vi "niLvFpga_AcknowledgeIrq_USB-7846R.vi"(0 "session in":u32, 5 "IRQ Numbers":i32[](array[numeric]), 11 "error in":errorcluster) -> (4 "session out":u32, 15 "error out":errorcluster)   [LabVIEW 2020]
uses:
  <vilib>/rvi/interface/common/niFpgaWaitOnOcc.vi
  NiFpgaLv.dll
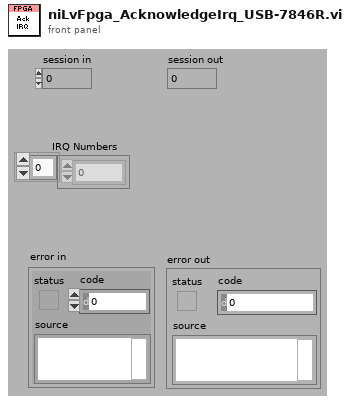
[diagram p1: front panel]
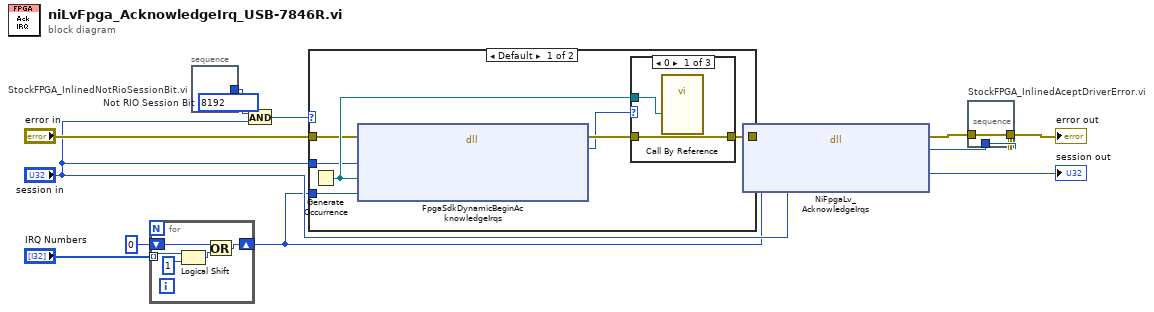
[diagram p0: block diagram]
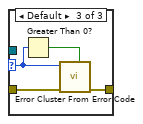
[diagram p4: hidden frame]
diagram:
  n1 = for {
    tunnel: "IRQ Numbers" -> [w16] mode=indexing
    shift-right: [w13] -> w1
    shift-left: u32 0 -> [w15]
    n2 = Logical Shift(y=w16, x=u32 1) -> (x << y=w14:u32)
    n3 = Or(x=w15, y=w14) -> (x .or. y?=w13:u32)
  }
  n4 = stacked-sequence "StockFPGA_InlinedNotRioSessionBit.vi" {
    tunnel: [w18] -> w6
    frame #0 {
      w18 = u32 8192  # Not RIO Session Bit
    }
  }
  n5 = And(x=w6, y="session in") -> (x .and. y?=w5:u32)
  n6 = case shown="Default" w5 {
    tunnel: "error in" -> [w22 w33]
    tunnel: [w21 w33] -> w3
    tunnel: "session in" -> [w20 _]
    tunnel: w1 -> [w19 _]
    frame Default {
      n7 = Generate Occurrence() -> (w25:refnum<k4>)
      n8 = dll-call lib="LabVIEW" fn="FpgaSdkDynamicBeginAcknowledgeIrqs" label="BeginAcknowledgeIrqs"(error in=w22, "session"=w20, "occurrence"=w25, "irqMask"=w19) -> (error out=w24:errorcluster, "status"=w23:i32)  [unwired: 5 in, 1 out]
      n9 = case shown="0" w23 {
        selector: w23 -> [_ _ w29]
        tunnel: [w27 w28 w31] -> w21
        tunnel: w24 -> [w27 w28 w32]
        tunnel: w25 -> [w26 _ _]
        frame 0 {
          n10 = call-by-ref "?"("occurrence"=w26) -> ()  [unwired: 16 in, 3 out]
        }
        frame -61167 {
          # "emulation case intentionally ignoring error"
        }
        frame Default {
          n11 = Greater Than 0?(x=w29) -> (x > 0?=w30:bool)
          n12 = call <vilib>:"Error Cluster From Error Code.vi"("is warning? (False)"=w30, "error in (no error)"=w32, "error code (0)"=w29) -> ("error out"=w31:errorcluster)  [unwired: 6 in]
        }
      }
    }
    frame 0 {
    }
  }
  n13 = dll-call lib="NiFpgaLv.*" fn="NiFpgaLv_AcknowledgeIrqs" label="niLvFpgaAcknowledgeIRQ"(error in=w3, "sessionID"="session in", "irqNumberMask"=w1) -> (error out=w11:errorcluster, "status"=w10:i32, "sessionID"=→"session out":u32)  [unwired: 3 in, 1 out]
  n14 = stacked-sequence "StockFPGA_InlinedAceptDriverError.vi" {
    tunnel: w11 -> [w34]
    tunnel: w10 -> [w36]
    tunnel: [w35] -> w12
    frame #0 {
      n15 = case shown="Default" w36 {
        selector: w36 -> [_ w38]
        tunnel: [w37 w40] -> w35
        tunnel: w34 -> [w37 w41]
        frame 0 {
        }
        frame Default {
          n16 = Greater Than 0?(x=w38) -> (x > 0?=w39:bool)
          n17 = call <vilib>:"Error Cluster From Error Code.vi"("is warning? (False)"=w39, "error in (no error)"=w41, "error code (0)"=w38) -> ("error out"=w40:errorcluster)  [unwired: 6 in]
        }
      }
    }
  }
  "error out" <- w12
